vi "pulse_generator_multiheater_continuous_driver_refnum.vi"(2 "Stop! Refnum":refnum<vi>, 3 "Pulse Generator Control Multiheater Refnums":T1) -> ()   [LabVIEW 2017]
uses:
  <vilib>/Utility/error.llb/DialogType.ctl
  <vilib>/DAQmx/write.llb/DAQmx Write (Digital 1D Bool NChan 1Samp 1Line).vi
  <vilib>/Instr/_visa.llb/VISA Configure Serial Port (Instr).vi
  <vilib>/DAQmx/create/channels.llb/DAQmx Create Channel (DO-Digital Output).vi
  pulse_generator_controls_multiheater_refnums.ctl
panel:
  out "error out":errorcluster
  out "Motor Error Code":string
  out "Stopped!":bool caption="OK"
  in  "Stop! Local":bool
  in  "SwitchHelper":bool
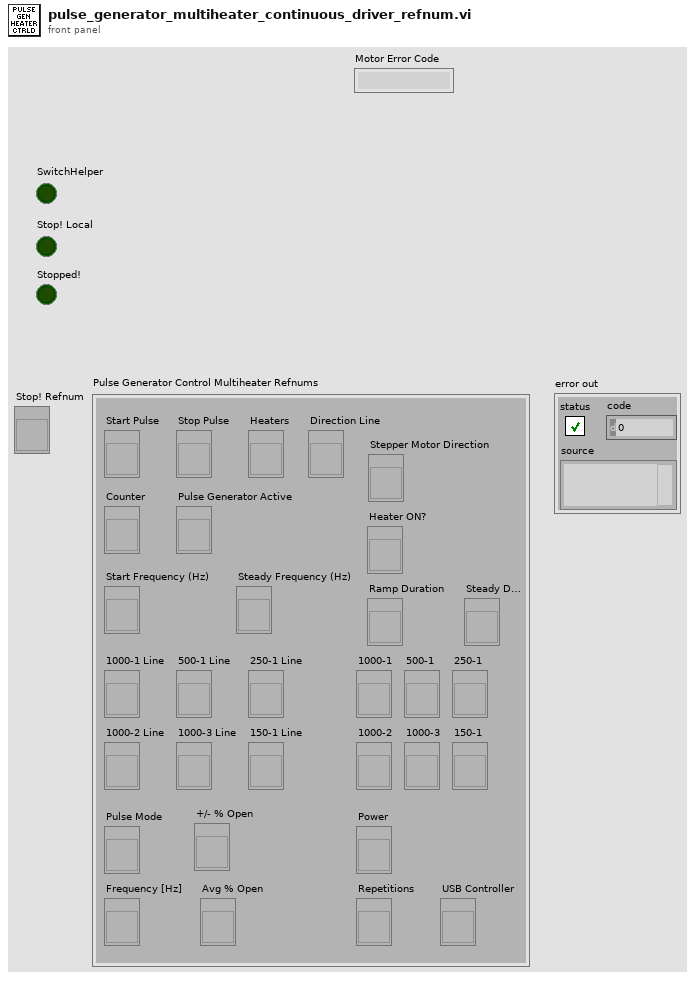
[diagram p1: front panel]
types:
  T1 = typedef "pulse_generator_controls_multiheater_refnums.ctl" = cluster{"Start Pulse":refnum<vi>, "Stop Pulse":refnum<vi>, "Heaters":refnum<vi>, "Counter":refnum<vi>, "Start Frequency (Hz)":refnum<vi>, "Pulse Generator Active":refnum<vi>, "Stepper Motor Direction":refnum<vi>, "Ramp Duration":refnum<vi>, "Direction Line":refnum<vi>, "1000-1 Line":refnum<vi>, "1000-2 Line":refnum<vi>, "1000-3 Line":refnum<vi>, "500-1 Line":refnum<vi>, "250-1 Line":refnum<vi>, "1000-1":refnum<vi>, "1000-2":refnum<vi>, "1000-3":refnum<vi>, "500-1":refnum<vi>, "250-1":refnum<vi>, "150-1":refnum<vi>, "Heater ON?":refnum<vi>, "150-1 Line":refnum<vi>, "Power":refnum<vi>, "Steady Frequency (Hz)":refnum<vi>, "Steady Duration ":refnum<vi>, "Pulse Mode":refnum<vi>, "Frequency [Hz]":refnum<vi>, "Avg % Open":refnum<vi>, "Repetitions":refnum<vi>, "+/- % Open":refnum<vi>, "USB Controller":refnum<vi>}
  T2 = enum8{"Enabled", "Disabled", "Disabled and Grayed Out"}
  T3 = typedef "DialogType.ctl" = u16
  T4 = cluster{"1000-1":refnum<vi>, "1000-2":refnum<vi>, "1000-3":refnum<vi>, "500-1":refnum<vi>, "250-1":refnum<vi>, "150-1":refnum<vi>}
  T5 = cluster{"1000-1 Line":refnum<vi>, "1000-2 Line":refnum<vi>, "1000-3 Line":refnum<vi>, "500-1 Line":refnum<vi>, "250-1 Line":refnum<vi>, "150-1 Line":refnum<vi>}
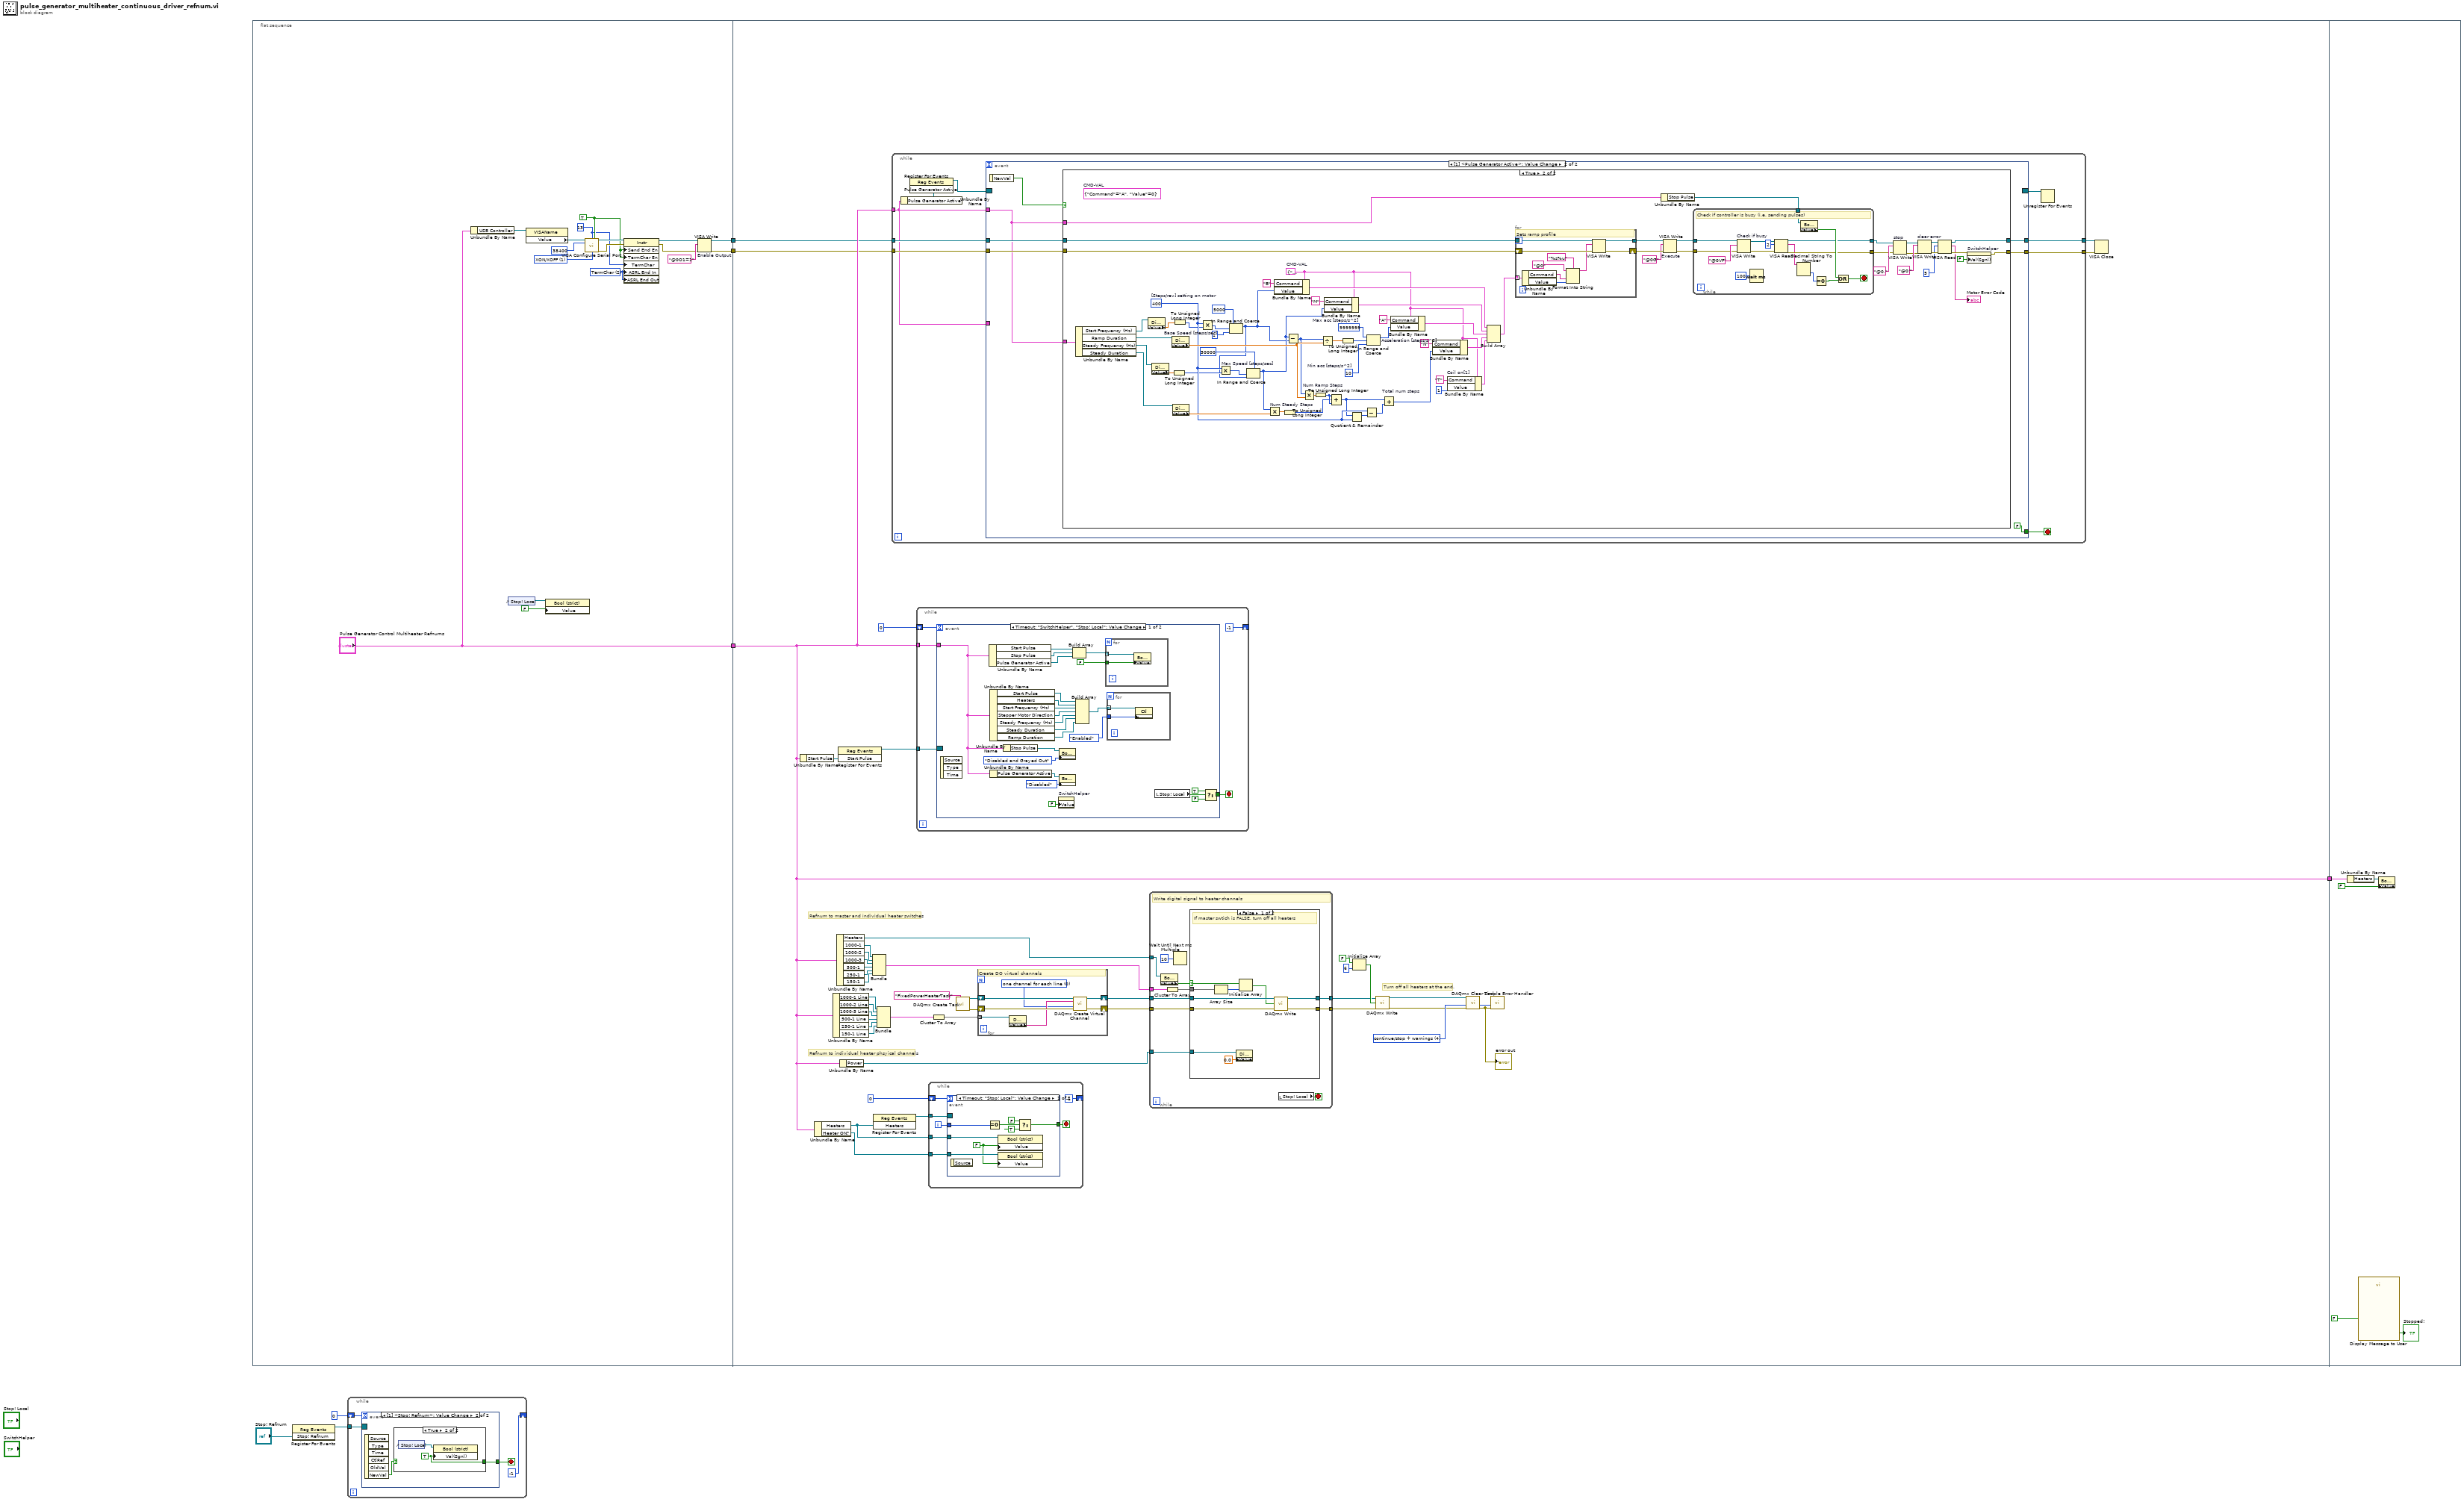
[diagram p0: block diagram]
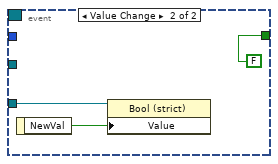
[diagram p2: hidden frame]
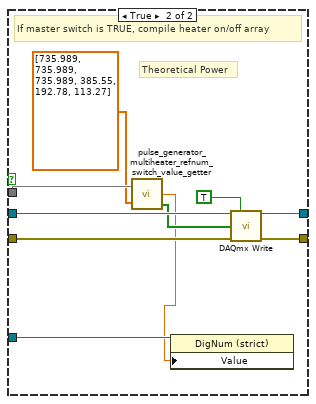
[diagram p3: hidden frame]
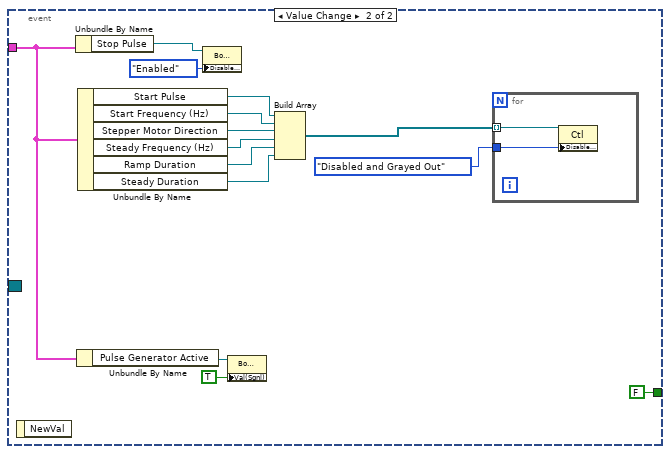
[diagram p4: hidden frame]
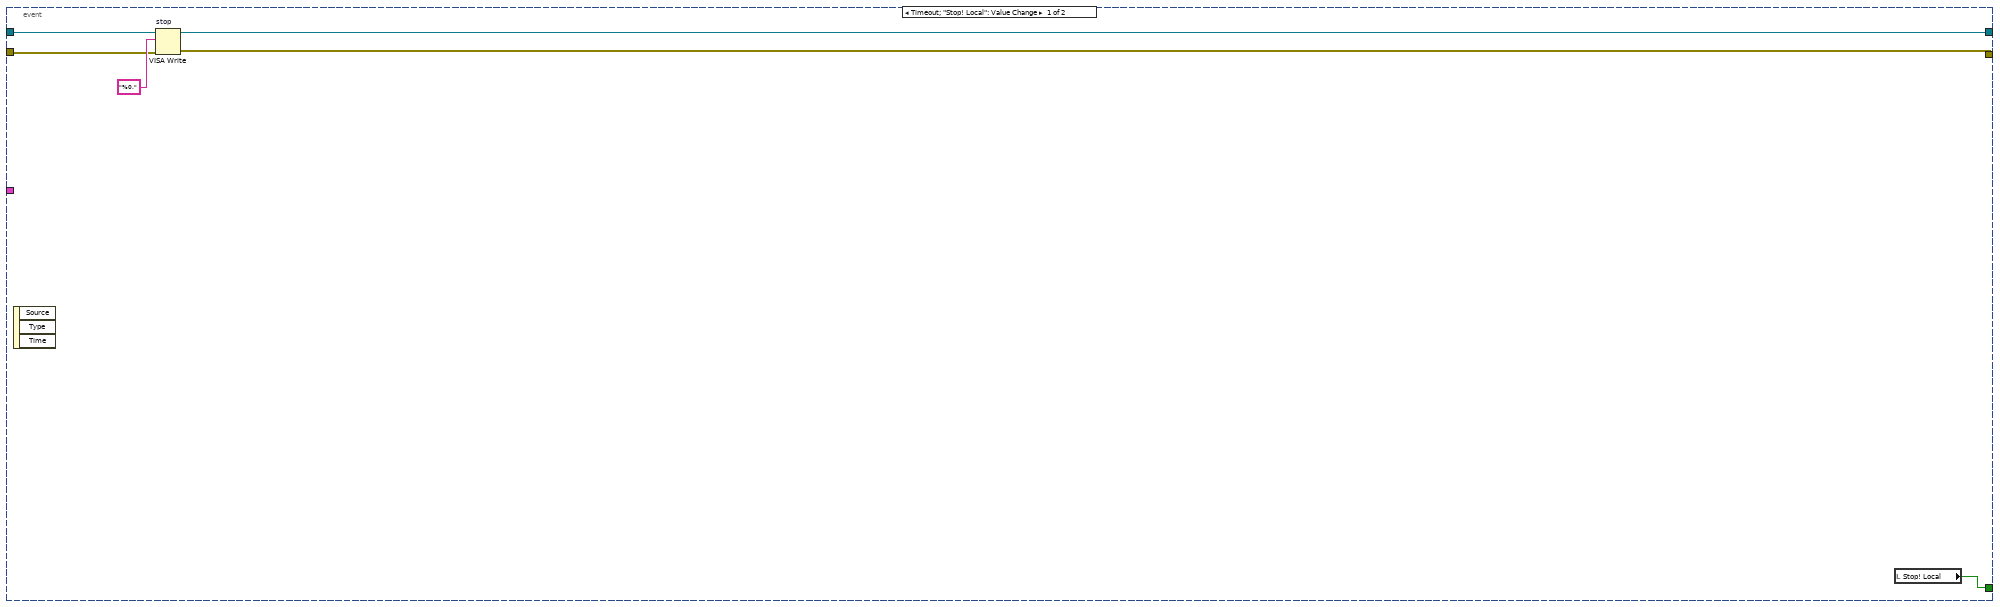
[diagram p5: hidden frame]
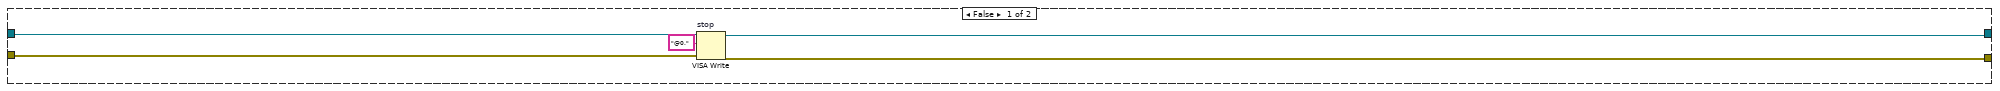
[diagram p6: hidden frame]
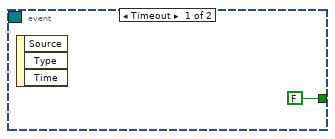
[diagram p7: hidden frame]
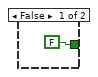
[diagram p8: hidden frame]
diagram:
  n1 = flat-sequence {
    tunnel: ["Pulse Generator Control Multiheater Refnums"] -> w3
    tunnel: [w9] -> w2
    tunnel: [w8] -> w1
    tunnel: [w29] -> w4
    tunnel: w3 -> [w29]
    tunnel: w2 -> [w28]
    tunnel: w1 -> [w27]
    tunnel: w4 -> [w296]
    frame #0 {
      w13 = u16 2 items=["None", "Last Bit", "TermChar"] ("Serial Settings:End Mode for Reads")
      w14 = u8 13 ("termination char\n(0xA = '\\n' = LF)")
      w15 = TRUE ("Enable Termination\nChar (T)")
      w20 = u16 1 items=["None", "XON/XOFF", "RTS/CTS", "XON/XOFF & RTS/CTS", "DTR/DSR", "XON/XOFF & DTR/DSR"] ("flow control (0:none)")
      n2 = Unbundle By Name("Pulse Generator Control Multiheater Refnums") -> ("USB Controller"=w16:refnum<vi>)
      n3 = control-ref of="Stop! Local"() -> (w23:refnum<vi>)
      n4 = property class="VISAName"(reference=w16) -> ("Value"=w18:refnum<visa-resource-name>)  [unwired: 1 in, 2 out]
      n5 = property class="Bool (strict)"(reference=w23, "Value"=FALSE) -> ()  [unwired: 1 in, 2 out]
      n6 = call-poly "VISA Configure Serial Port"("VISA resource name"=w18, "termination char\n(0xA = '\\n' = LF)"=w14, "Enable Termination\nChar (T)"=w15, "baud rate (9600)"=u32 38400, "flow control (0:none)"=w20) -> ("VISA resource name out"=w21:refnum<visa-resource-name>, "error out"=w22:errorcluster)  [unwired: 9 in]
      n7 = property class="Instr"(reference=w21, error in=w22, "Send End En"=w15, "TermChar En"=w15, "TermChar"=w14, "ASRL End In"=w13, "ASRL End Out"=w13) -> (reference out=w11:refnum<visa-resource-name>, error out=w10:errorcluster)
      n8 = VISA Write "Enable Output"(VISA resource name=w11, write buffer="@0O1=1", error in (no error)=w10) -> (VISA resource name out=w9:refnum<visa-resource-name>, error out=w8:errorcluster)  [unwired: 1 out]
    }
    frame #1 {
      w62 = T3 4 items=["no dialog", "OK message", "continue or stop message", "OK message + warnings", "continue/stop + warnings"] ("type of dialog (OK msg:1)")
      # "Turn off all heaters at the end."
      # "Refnum to individual heater phsyical channels"
      # "Refnum to master and individual heater switches"
      n9 = Unbundle By Name(w29) -> ("Start Pulse"=w65:refnum<vi>)
      n10 = Unbundle By Name(w29) -> ("Heaters"=w57:refnum<vi>, "Heater ON?"=w39:refnum<vi>)
      n11 = Unbundle By Name(w29) -> ("1000-1 Line"=w36:refnum<vi>, "1000-2 Line"=w35:refnum<vi>, "1000-3 Line"=w34:refnum<vi>, "500-1 Line"=w33:refnum<vi>, "250-1 Line"=w32:refnum<vi>, "150-1 Line"=w31:refnum<vi>)
      n12 = Unbundle By Name(w29) -> ("Heaters"=w56:refnum<vi>, "1000-1"=w55:refnum<vi>, "1000-2"=w54:refnum<vi>, "1000-3"=w53:refnum<vi>, "500-1"=w52:refnum<vi>, "250-1"=w50:refnum<vi>, "150-1"=w40:refnum<vi>)
      n13 = register-events(w65) -> (reference out=w66:refnum<event-registration>)  [unwired: 2 in, 1 out]
      n14 = Unbundle By Name(w29) -> ("Power"=w30:refnum<vi>)
      n15 = Bundle("1000-1"=w55, "1000-2"=w54, "1000-3"=w53, "500-1"=w52, "250-1"=w50, "150-1"=w40) -> (w37:T4)  [unwired: 1 in]
      n16 = register-events(w57) -> (reference out=w61:refnum<event-registration>)  [unwired: 2 in, 1 out]
      n17 = Bundle("1000-1 Line"=w36, "1000-2 Line"=w35, "1000-3 Line"=w34, "500-1 Line"=w33, "250-1 Line"=w32, "150-1 Line"=w31) -> (w38:T5)  [unwired: 1 in]
      n18 = while {
        tunnel: w29 -> [w175]
        tunnel: w28 -> [w177]
        tunnel: w27 -> [w176]
        tunnel: [w174] -> w26
        tunnel: [w173] -> w25
        stop <- w180 stop-if-true
        n19 = Unbundle By Name(w175) -> ("Pulse Generator Active"=w179:refnum<vi>)
        n20 = register-events(w179) -> (reference out=w181:refnum<event-registration>)  [unwired: 2 in, 1 out]
        n21 = event shown="[1] <Pulse Generator Active>: Value Change" {
          selector: w181 -> [_ _]
          dyn-events: [_ _] -> w178
          timeout: _ -> [_ _]
          tunnel: [w187 FALSE ("Stop! Local")] -> w180
          tunnel: w175 -> [_ _]
          tunnel: w177 -> [w185 w192]
          tunnel: w176 -> [w184 w191]
          tunnel: w175 -> [_ w188]
          tunnel: [w183 w190] -> w174
          tunnel: [w182 w189] -> w173
          event Timeout; "Stop! Local": Value Change {
            n22 = event-data() -> ()  [unwired: 1 in, 3 out]
            n23 = VISA Write "stop"(VISA resource name=w185, write buffer="%0.", error in (no error)=w184) -> (VISA resource name out=w183:refnum<visa-resource-name>, error out=w182:errorcluster)  [unwired: 1 out]
            n24 = local read "Stop! Local"() -> (w187:bool)
          }
          event Value Change {
            n25 = event-data() -> ("NewVal"=w193:bool)  [unwired: 1 in]
            n26 = case shown="True" w193 {
              tunnel: w188 -> [_ w264]
              tunnel: w192 -> [w198 w254]
              tunnel: w191 -> [w197 w253]
              tunnel: [w196 w202] -> w190
              tunnel: [w195 w213] -> w189
              tunnel: w188 -> [_ w217]
              frame False {
                n27 = VISA Write "stop"(VISA resource name=w198, write buffer="@0.", error in (no error)=w197) -> (VISA resource name out=w196:refnum<visa-resource-name>, error out=w195:errorcluster)  [unwired: 1 out]
              }
              frame True {
                w218 = cluster{"Command":string, "Value":u32} {"Command"="A", "Value"=0}  # CMD-VAL
                (unwired) cluster{"Command":string, "Value":u32} {"Command"="A", "Value"=0}  # CMD-VAL
                w261 = u32 9999999  # Max acc [steps/s^2]
                w263 = u32 10  # Min acc [steps/s^2]
                w256 = u32 400  # [Steps/rev] setting on motor
                n28 = Unbundle By Name(w264) -> ("Start Frequency (Hz)"=w267:refnum<vi>, "Ramp Duration"=w265:refnum<vi>, "Steady Frequency (Hz)"=w266:refnum<vi>, "Steady Duration"=w268:refnum<vi>)
                n29 = property class="DigNum (strict)"(reference=w267) -> ("Value"=w236:dbl)  [unwired: 1 in, 2 out]
                n30 = property class="DigNum (strict)"(reference=w266) -> ("Value"=w234:dbl)  [unwired: 1 in, 2 out]
                n31 = property class="DigNum (strict)"(reference=w265) -> ("Value"=w258:dbl)  [unwired: 1 in, 2 out]
                n32 = property class="DigNum (strict)"(reference=w268) -> ("Value"=w259:dbl)  [unwired: 1 in, 2 out]
                n33 = To Unsigned Long Integer(number=w234) -> (unsigned 32bit integer=w233:u32)
                n34 = To Unsigned Long Integer(number=w236) -> (unsigned 32bit integer=w235:u32)
                n35 = Multiply "Base Speed [steps/sec]"(x=w256, y=w235) -> (x*y=w238:u32)
                n36 = Multiply "Max Speed [steps/sec]"(x=w256, y=w233) -> (x*y=w241:u32)
                n37 = In Range and Coerce(upper limit=u32 5000, x=w238, lower limit=u32 1) -> (coerced(x)=w230:u32)  [unwired: 1 out]
                n38 = In Range and Coerce(upper limit=u32 50000, x=w241, lower limit=w230) -> (coerced(x)=w239:u32)  [unwired: 1 out]
                n39 = Multiply "Num Steady Steps"(x=w239, y=w259) -> (x*y=w227:dbl)
                n40 = Bundle By Name(cluster=w218, "Command"="B", "Value"=w230) -> (w243:cluster{"Command":string, "Value":u32})
                n41 = To Unsigned Long Integer(number=w227) -> (unsigned 32bit integer=w226:u32)
                n42 = Subtract(x=w239, y=w230) -> (x-y=w231:u32)
                n43 = Multiply "Num Ramp Steps"(x=w231, y=w258) -> (x*y=w229:dbl)
                n44 = To Unsigned Long Integer(number=w229) -> (unsigned 32bit integer=w228:u32)
                n45 = Divide(x=w231, y=w258) -> (x/y=w260:dbl)
                n46 = Bundle By Name(cluster=w218, "Command"="M", "Value"=w239) -> (w244:cluster{"Command":string, "Value":u32})
                n47 = Compound Arithmetic op=ADD(w228, w226, w228) -> (w225:u32)
                n48 = To Unsigned Long Integer(number=w260) -> (unsigned 32bit integer=w262:u32)
                n49 = Quotient & Remainder(x=w225, y=w256) -> (x-y*floor(x/y)=w257:u32)  [unwired: 1 out]
                n50 = Subtract(x=w256, y=w257) -> (x-y=w255:u32)
                n51 = In Range and Coerce "Acceleration [steps/s^2]"(upper limit=w261, x=w262, lower limit=w263) -> (coerced(x)=w250:u32)  [unwired: 1 out]
                n52 = Add "Total num steps"(x=w225, y=w255) -> (x+y=w247:u32)
                n53 = Bundle By Name(cluster=w218, "Command"="A", "Value"=w250) -> (w245:cluster{"Command":string, "Value":u32})
                n54 = Bundle By Name(cluster=w218, "Command"="N", "Value"=w247) -> (w246:cluster{"Command":string, "Value":u32})
                n55 = Bundle By Name "Coil on[1]"(cluster=w218, "Command"="T", "Value"=u32 1) -> (w219:cluster{"Command":string, "Value":u32})
                n56 = Build Array(w243, w244, w245, w246, w219) -> (w242:cluster{"Command":string, "Value":u32}[])
                n57 = for {
                  tunnel: w254 -> [w293]
                  tunnel: w242 -> [w291] mode=indexing
                  tunnel: [w285] -> w224
                  shift-right: [w284] -> w223
                  shift-left: w253 -> [w292]
                  # "Sets ramp profile"
                  n58 = Unbundle By Name(w291) -> ("Command"=w289:string, "Value"=w290:u32)
                  n59 = Format Into String(format string="%s%u", initial string="@0" ("format string"), w289, w290) -> (resulting string=w287:string)  [unwired: 1 in, 1 out]
                  n60 = VISA Write(VISA resource name=w293, write buffer=w287, error in (no error)=w292) -> (VISA resource name out=w285:refnum<visa-resource-name>, error out=w284:errorcluster)  [unwired: 1 out]
                }
                n61 = Unbundle By Name(w217) -> ("Stop Pulse"=w214:refnum<vi>)
                n62 = VISA Write "Execute"(VISA resource name=w224, write buffer="@0G", error in (no error)=w223) -> (VISA resource name out=w216:refnum<visa-resource-name>, error out=w215:errorcluster)  [unwired: 1 out]
                n63 = while {
                  tunnel: w216 -> [w281]
                  tunnel: w215 -> [w282]
                  tunnel: w214 -> [w276]
                  tunnel: [w272] -> w210
                  tunnel: [w271] -> w209
                  stop <- w273 stop-if-true
                  # "Check if controller is busy (i.e. sending pulses)"
                  n64 = VISA Write "Check if busy"(VISA resource name=w281, write buffer="@0VF", error in (no error)=w282) -> (VISA resource name out=w280:refnum<visa-resource-name>, error out=w279:errorcluster)  [unwired: 1 out]
                  n65 = Wait (ms)(milliseconds to wait=u32 100) -> ()  [unwired: 1 out]
                  n66 = VISA Read(VISA resource name=w280, byte count=u32 2, error in (no error)=w279) -> (VISA resource name out=w272:refnum<visa-resource-name>, read buffer=w269:string, error out=w271:errorcluster)  [unwired: 1 out]
                  n67 = Decimal String To Number(string=w269) -> (number=w277:i32)  [unwired: 2 in, 1 out]
                  n68 = property class="Bool (strict)"(reference=w276) -> ("Value"=w274:bool)  [unwired: 1 in, 2 out]
                  n69 = Equal To 0?(x=w277) -> (x = 0?=w275:bool)
                  n70 = Compound Arithmetic op=OR(w274, w275) -> (w273:bool)
                }
                n71 = VISA Write "stop"(VISA resource name=w210, write buffer="@0.", error in (no error)=w209) -> (VISA resource name out=w207:refnum<visa-resource-name>, error out=w206:errorcluster)  [unwired: 1 out]
                n72 = VISA Write "clear error"(VISA resource name=w207, write buffer="@0!", error in (no error)=w206) -> (VISA resource name out=w204:refnum<visa-resource-name>, error out=w205:errorcluster)  [unwired: 1 out]
                n73 = VISA Read(VISA resource name=w204, byte count=u32 5, error in (no error)=w205) -> (VISA resource name out=w202:refnum<visa-resource-name>, read buffer=→"Motor Error Code":string, error out=w201:errorcluster)  [unwired: 1 out]
                n74 = property on="SwitchHelper" class="Bool (strict)"(error in=w201, "Val(Sgnl)"=FALSE ("Value (Signaling)")) -> (error out=w213:errorcluster)  [unwired: 1 in, 1 out]
              }
            }
          }
        }
        n75 = Unregister For Events(event registration refnum=w178) -> ()  [unwired: 1 in, 1 out]
      }
      n76 = while {
        shift-right: [-1] -> _
        shift-left: 0 -> [w128]
        tunnel: w66 -> [w126]
        tunnel: w29 -> [w124]
        stop <- w125 stop-if-true
        n77 = event shown="[0] Timeout;  \"SwitchHelper\", \"Stop! Local\": Value Change" {
          selector: w126 -> [_ _]
          dyn-events: _ -> [_ _]
          timeout: w128 -> [_ _]
          tunnel: [w149 FALSE ("Value")] -> w125
          tunnel: w124 -> [w131 w159]
          event Timeout; "SwitchHelper", "Stop! Local": Value Change {
            n78 = event-data() -> ()  [unwired: 1 in, 3 out]
            n79 = Unbundle By Name(w131) -> ("Start Pulse"=w138:refnum<vi>, "Stop Pulse"=w137:refnum<vi>, "Pulse Generator Active"=w136:refnum<vi>)
            n80 = Unbundle By Name(w131) -> ("Start Pulse"=w142:refnum<vi>, "Heaters"=w146:refnum<vi>, "Start Frequency (Hz)"=w145:refnum<vi>, "Stepper Motor Direction"=w144:refnum<vi>, "Steady Frequency (Hz)"=w143:refnum<vi>, "Steady Duration"=w130:refnum<vi>, "Ramp Duration"=w129:refnum<vi>)
            n81 = Unbundle By Name(w131) -> ("Pulse Generator Active"=w134:refnum<vi>)
            n82 = Unbundle By Name(w131) -> ("Stop Pulse"=w133:refnum<vi>)
            n83 = property on="SwitchHelper" class="Bool (strict)"("Value"=FALSE) -> ()  [unwired: 2 in, 2 out]
            n84 = property class="Bool (strict)"(reference=w133, "DisabledEnum"=T2."Disabled and Grayed Out" ("Disabled")) -> ()  [unwired: 1 in, 2 out]
            n85 = property class="Bool (strict)"(reference=w134, "DisabledEnum"=T2."Disabled" ("Disabled")) -> ()  [unwired: 1 in, 2 out]
            n86 = Build Array(w138, w137, w136) -> (w139:refnum<vi>[])
            n87 = Build Array(w142, w146, w145, w144, w143, w130, w129) -> (w141:refnum<vi>[])
            n88 = for {
              tunnel: w139 -> [w154] mode=indexing
              tunnel: FALSE ("Value") -> [w153]
              n89 = property class="Bool (strict)"(reference=w154, "Value"=w153) -> ()  [unwired: 1 in, 2 out]
            }
            n90 = for {
              tunnel: w141 -> [w156] mode=indexing
              tunnel: T2."Enabled" ("Disabled") -> [w155]
              n91 = property class="Ctl"(reference=w156, "DisabledEnum"=w155) -> ()  [unwired: 1 in, 2 out]
            }
            n92 = local read "Stop! Local"() -> (w150:bool)
            n93 = Select(t=TRUE ("Value"), s=w150, f=FALSE ("Value")) -> (s? t:f=w149:bool)
          }
          event Value Change {
            n94 = event-data() -> ()  [unwired: 1 in, 1 out]
            n95 = Unbundle By Name(w159) -> ("Stop Pulse"=w163:refnum<vi>)
            n96 = Unbundle By Name(w159) -> ("Pulse Generator Active"=w161:refnum<vi>)
            n97 = Unbundle By Name(w159) -> ("Start Pulse"=w166:refnum<vi>, "Start Frequency (Hz)"=w167:refnum<vi>, "Stepper Motor Direction"=w168:refnum<vi>, "Steady Frequency (Hz)"=w169:refnum<vi>, "Ramp Duration"=w158:refnum<vi>, "Steady Duration"=w157:refnum<vi>)
            n98 = property class="Bool (strict)"(reference=w163, "DisabledEnum"=T2."Enabled" ("Disabled")) -> ()  [unwired: 1 in, 2 out]
            n99 = property class="Bool (strict)"(reference=w161, "Val(Sgnl)"=TRUE ("Value")) -> ()  [unwired: 1 in, 2 out]
            n100 = Build Array(w166, w167, w168, w169, w158, w157) -> (w165:refnum<vi>[])
            n101 = for {
              tunnel: w165 -> [w172] mode=indexing
              tunnel: T2."Disabled and Grayed Out" ("Disabled") -> [w171]
              n102 = property class="Ctl"(reference=w172, "DisabledEnum"=w171) -> ()  [unwired: 1 in, 2 out]
            }
          }
        }
      }
      n103 = while {
        tunnel: w61 -> [w81]
        shift-right: [-1 ("millisecond multiple")] -> _
        shift-left: 0 ("millisecond multiple") -> [w80]
        tunnel: w57 -> [w78]
        tunnel: w39 -> [w75]
        i -> [w77]
        stop <- w76 stop-if-true
        n104 = event shown="[0] Timeout;  \"Stop! Local\": Value Change" {
          selector: w81 -> [_ _]
          dyn-events: _ -> [_ _]
          timeout: w80 -> [_ _]
          tunnel: w78 -> [w89 _]
          tunnel: w77 -> [w87 _]
          tunnel: [w84 FALSE ("f")] -> w76
          tunnel: w75 -> [w83 w90]
          event Timeout; "Stop! Local": Value Change {
            w82 = FALSE ("Value")
            n105 = event-data() -> ()  [unwired: 1 in, 1 out]
            n106 = Equal To 0?(x=w87) -> (x = 0?=w88:bool)
            n107 = property class="Bool (strict)"(reference=w89, "Value"=w82) -> ()  [unwired: 1 in, 2 out]
            n108 = property class="Bool (strict)"(reference=w83, "Value"=w82) -> ()  [unwired: 1 in, 2 out]
            n109 = Select(t=FALSE, s=w88, f=TRUE) -> (s? t:f=w84:bool)
          }
          event Value Change {
            n110 = event-data() -> ("NewVal"=w91:bool)  [unwired: 1 in]
            n111 = property class="Bool (strict)"(reference=w90, "Value"=w91) -> ()  [unwired: 1 in, 2 out]
          }
        }
      }
      n112 = Cluster To Array(cluster=w38) -> (array=w51:refnum<vi>[])
      n113 = call <vilib>:"DAQmx Create Task.vi"("new task name"="FixedPowerHeaterTask") -> ("task out"=w60:refnum<k21>, "error out"=w59:errorcluster)  [unwired: 13 in]
      n114 = for {
        tunnel: w51 -> [w70] mode=indexing
        shift-right: [w74] -> w43
        shift-left: w60 -> [w72]
        shift-right: [w73] -> w42
        shift-left: w59 -> [w71]
        w68 = 0 items=["one channel for each line", "one channel for all lines"] ("line grouping")
        # "Create DO virtual channels"
        n115 = property class="DAQmxName"(reference=w70) -> ("Value"=w69:string)  [unwired: 1 in, 2 out]
        n116 = call-poly <vilib>:"DAQmx Create Virtual Channel.vi"("task in"=w72, "lines"=w69, "line grouping"=w68, "error in"=w71) -> ("task out"=w74:refnum<k21>, "error out"=w73:errorcluster)  [unwired: 10 in]
      }
      n117 = while {
        tunnel: w43 -> [w101]
        tunnel: w42 -> [w100]
        tunnel: w56 -> [w97]
        tunnel: [w99] -> w45
        tunnel: [w98] -> w44
        tunnel: w37 -> [w95]
        tunnel: w30 -> [w93]
        stop <- w102 stop-if-true
        # "Write digital signal to heater channels"
        n118 = property class="Bool (strict)"(reference=w97) -> ("Value"=w96:bool)  [unwired: 1 in, 2 out]
        n119 = Cluster To Array(cluster=w95) -> (array=w94:refnum<vi>[])
        n120 = Wait Until Next ms Multiple(millisecond multiple=u32 10) -> ()  [unwired: 1 out]
        n121 = case shown="False" w96 {
          selector: w96 -> [w106 _]
          tunnel: w101 -> [w113 w122]
          tunnel: w100 -> [w112 w121]
          tunnel: [w110 w123] -> w99
          tunnel: [w111 w120] -> w98
          tunnel: w94 -> [w108 w118]
          tunnel: w93 -> [w105 w115]
          frame False {
            # "If master swtich is FALSE, turn off all heaters"
            n122 = Array Size(array=w108) -> (size(s)=w109:i32)
            n123 = property class="DigNum (strict)"(reference=w105, "Value"=0.0) -> ()  [unwired: 1 in, 2 out]
            n124 = Initialize Array(w106, w109) -> (w107:bool[])
            n125 = call-poly <vilib>:"DAQmx Write.vi"("task/channels in"=w113, "data"=w107, "error in"=w112) -> ("task out"=w110:refnum<k21>, "error out"=w111:errorcluster)  [unwired: 10 in, 1 out]
          }
          frame True {
            # "Theoretical Power"
            # "If master switch is TRUE, compile heater on/off array"
            n126 = call "pulse_generator_multiheater_refnum_switch_value_getter.vi"("On/Off Refnums"=w118, "Power Array"=dbl[] [735.989, 735.989, 735.989, 385.55, 192.78, 113.27]) -> ("Total Power"=w114:dbl, "Digital"=w117:bool[])  [unwired: 1 out]
            n127 = property class="DigNum (strict)"(reference=w115, "Value"=w114) -> ()  [unwired: 1 in, 2 out]
            n128 = call-poly <vilib>:"DAQmx Write.vi"("task/channels in"=w122, "auto start"=TRUE, "data"=w117, "error in"=w121) -> ("task out"=w123:refnum<k21>, "error out"=w120:errorcluster)  [unwired: 9 in, 1 out]
          }
        }
        n129 = local read "Stop! Local"() -> (w102:bool)
      }
      n130 = Initialize Array(FALSE ("element"), 6 ("dimension size")) -> (w46:bool[])
      n131 = call-poly <vilib>:"DAQmx Write.vi"("task/channels in"=w45, "data"=w46, "error in"=w44) -> ("task out"=w49:refnum<k21>, "error out"=w48:errorcluster)  [unwired: 10 in, 1 out]
      n132 = call <vilib>:"DAQmx Clear Task.vi"("task in"=w49, "error in"=w48) -> ("error out"=w64:errorcluster)  [unwired: 13 in]
      "error out" <- w64
      n133 = call <vilib>:"Simple Error Handler.vi"("type of dialog (OK msg:1)"=w62, "error in (no error)"=w64) -> ()  [unwired: 3 in, 5 out]
      n134 = VISA Close(VISA resource name=w26, error in (no error)=w25) -> ()  [unwired: 1 out]
    }
    frame #2 {
      n135 = Unbundle By Name(w296) -> ("Heaters"=w295:refnum<vi>)
      n136 = call "Display Message to User"("Enable"=FALSE) -> ("OK"=→"Stopped!":bool)  [unwired: 9 in, 1 out]
      n137 = property class="Bool (strict)"(reference=w295, "Value"=FALSE) -> ()  [unwired: 1 in, 2 out]
    }
  }
  n138 = register-events("Stop! Refnum") -> (reference out=w6:refnum<event-registration>)  [unwired: 2 in, 1 out]
  n139 = while {
    tunnel: w6 -> [w302]
    shift-right: [-1] -> _
    shift-left: 0 -> [w301]
    stop <- w299 stop-if-true
    n140 = event shown="[1] <Stop! Refnum>: Value Change" {
      selector: w302 -> [_ _]
      dyn-events: _ -> [_ _]
      timeout: w301 -> [_ _]
      tunnel: [FALSE ("Value (Signaling)") w304] -> w299
      event Timeout {
        n141 = event-data() -> ()  [unwired: 1 in, 3 out]
      }
      event Value Change {
        n142 = event-data() -> ("NewVal"=w305:bool)  [unwired: 1 in, 5 out]
        n143 = case shown="True" w305 {
          tunnel: [FALSE ("Value (Signaling)") w308] -> w304
          frame False {
          }
          frame True {
            w308 = TRUE ("Value (Signaling)")
            n144 = control-ref of="Stop! Local"() -> (w307:refnum<vi>)
            n145 = property class="Bool (strict)"(reference=w307, "Val(Sgnl)"=w308) -> ()  [unwired: 1 in, 2 out]
          }
        }
      }
    }
  }
